vi "Read for Get Command.vi"(8 "error in (no error)":errorcluster, 10 "Control Name":string, 11 "TCP Network Connection in":refnum<k5>) -> (0 "error out":errorcluster)   [LabVIEW 2019]
doc: "Author: Scott Hannahs <sth@magnet.fsu.edu>\nCopyright 2018 Florida State University, All rights reserved."
uses:
  SCH Data Controls/FPGA Magnet Config.ctl
  SCH Data Controls/SCH Data 2 RT.ctl
  <vilib>/Utility/error.llb/Error Cluster From Error Code.vi
  TCP Functions/TCP Read Length and Value (I16).vi
  TCP Functions/TCP Read Length and Value (U16).vi
  TCP Functions/TCP Read Length and Value (I32).vi
  TCP Functions/TCP Read Length and Value (U32).vi
  TCP Functions/TCP Read Length and Value (Double).vi
  TCP Functions/TCP Read Length and Value (STR).vi
  TCP Functions/TCP Read Length and Value (Bool).vi
  TCP Functions/TCP Read Length and Value (DateStamp).vi
  TCP Functions/TCP Read Length and Value (Variant).vi
  TCP Functions/TCP Read Length and Value (Array I16).vi
  TCP Functions/TCP Read Length and Value (Array Dbl).vi
  TCP Functions/TCP Read Length and Value (2D Array Dbl).vi
  <vilib>/ErrorRing/Error Ring.xnode
  <vilib>/Utility/Data Type/NI_Data Type.lvlib
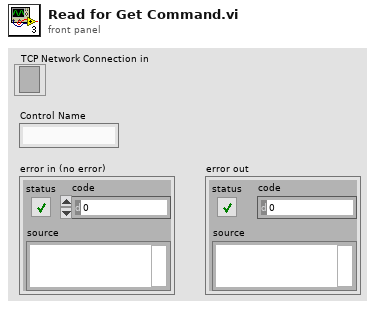
[diagram p1: front panel]
types:
  T1 = typedef "NI_Data Type.lvlib/Data Type.ctl" = enum8{"Invalid Type", "Void", "I8", "I16", "I32", "I64", "U8", "U16", "U32", "U64", "Single Float", "Double Float", "Extended Float", "Single Complex", "Double Complex", "Extended Complex", "Enum U8", "Enum U16", "Enum U32", "Enum U64", "Single Float With Unit", "Double Float With Unit", "Extended Float With Unit", "Single Complex with Unit", "Double Complex with Unit", "Extended Complex with Unit", "Boolean", "String", "Path", "Picture", "Tag", "Array", "Cluster", "Variant", "LV Variant", "Waveform", "Timestamp", "Digital Waveform", "Digital Data", "ExpressData", "Refnum", "External Data", "VI", "Poly VI", "LabVIEW Class Instance", "Fixed Point", "Set Collection", "Map Collection"}
  T2 = typedef "FPGA Magnet Config.ctl" = cluster{"#Coils":u32, "Coil Inductances":T3[], "Max Coil Currents":T3[], "Max Coil Volt Dev":T3[], "Coil A Coefficients":T3[], "Coil B Coefficients":T3[], "Coil C Coefficients":T3[], "Coil D Coefficients":T3[], "Max Coil Temp":T3[], " Pressure Range":T3[], "Temp Coef":T3[], "Offsets":T3[], "Scale Factors":T3[]}
  T3 = typedef "SCH Data 2 RT.ctl" = fxp<+/-,38,12>
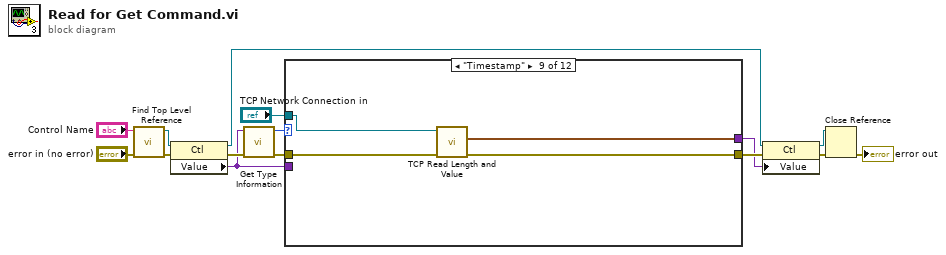
[diagram p0: block diagram]
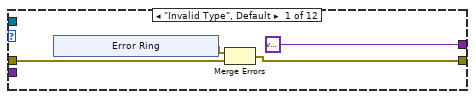
[diagram p2: hidden frame]
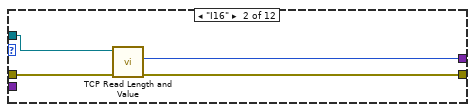
[diagram p3: hidden frame]
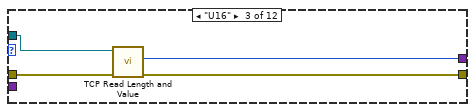
[diagram p4: hidden frame]
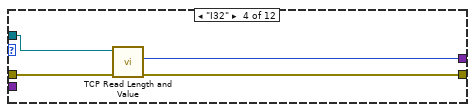
[diagram p5: hidden frame]
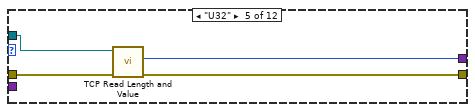
[diagram p6: hidden frame]
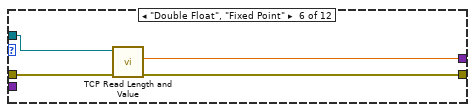
[diagram p7: hidden frame]
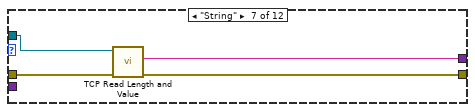
[diagram p8: hidden frame]
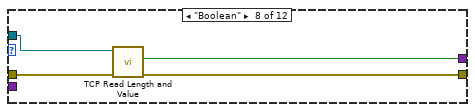
[diagram p9: hidden frame]
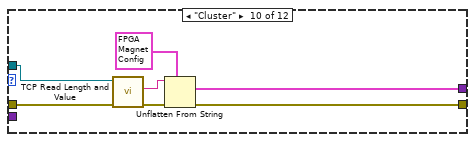
[diagram p10: hidden frame]
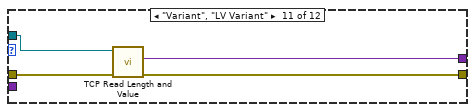
[diagram p11: hidden frame]
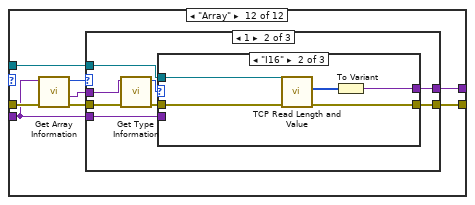
[diagram p12: hidden frame]
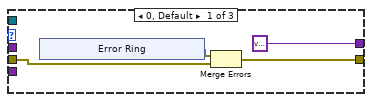
[diagram p13: hidden frame]
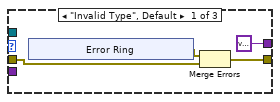
[diagram p14: hidden frame]
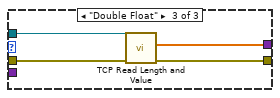
[diagram p15: hidden frame]
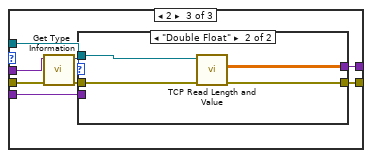
[diagram p16: hidden frame]
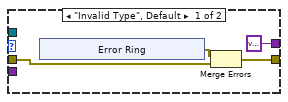
[diagram p17: hidden frame]
diagram:
  n1 = call "Find Top Level Reference.vi"("error in (no error)"="error in (no error)", "String"="Control Name") -> ("error out"=w11:errorcluster, "Ctl Refnum"=w10:refnum<vi>)  [unwired: 8 in]
  n2 = property class="Ctl"(reference=w10, error in=w11) -> (reference out=w1:refnum<vi>, error out=w12:errorcluster, "Value"=w5:variant)
  n3 = call <vilib>:"Get Type Information.vi"("error in (no error)"=w12, "variant"=w5) -> ("error out"=w6:errorcluster, "type"=w7:T1)  [unwired: 5 in, 3 out]
  n4 = case shown="\"Timestamp\"" w7 {
    tunnel: w5 -> [_ _ _ _ _ _ _ _ _ _ _ w69]
    tunnel: "TCP Network Connection in" -> [_ w26 w29 w36 w38 w43 w45 w50 w54 w63 w65 w75]
    tunnel: w6 -> [w19 w25 w32 w33 w37 w41 w46 w49 w53 w59 w64 w71]
    tunnel: [w18 w28 w31 w34 w40 w44 w47 w52 w56 w57 w67 w74] -> w3
    tunnel: [variant ("Variant") w27 w30 w35 w39 w42 w48 w51 w55 w60 w66 w68] -> w2
    frame "Invalid Type", Default {
      n5 = xnode "Error Ring"() -> ("error out"=w17:errorcluster)
      n6 = Merge Errors(w17, w19) -> (w18:errorcluster)
    }
    frame "I16" {
      n7 = call-poly "TCP Read Length and Value.vi"("error in (no error)"=w25, "TCP Network Connection in"=w26) -> ("error out"=w28:errorcluster, "Output"=w27:i16)  [unwired: 7 in, 1 out]
    }
    frame "U16" {
      n8 = call-poly "TCP Read Length and Value.vi"("error in (no error)"=w32, "TCP Network Connection in"=w29) -> ("error out"=w31:errorcluster, "Output"=w30:u16)  [unwired: 7 in, 1 out]
    }
    frame "I32" {
      n9 = call-poly "TCP Read Length and Value.vi"("error in (no error)"=w33, "TCP Network Connection in"=w36) -> ("error out"=w34:errorcluster, "Output"=w35:i32)  [unwired: 7 in, 1 out]
    }
    frame "U32" {
      n10 = call-poly "TCP Read Length and Value.vi"("error in (no error)"=w37, "TCP Network Connection in"=w38) -> ("error out"=w40:errorcluster, "Output"=w39:u32)  [unwired: 7 in, 1 out]
    }
    frame "Double Float", "Fixed Point" {
      n11 = call-poly "TCP Read Length and Value.vi"("error in (no error)"=w41, "TCP Network Connection in"=w43) -> ("error out"=w44:errorcluster, "Output"=w42:dbl)  [unwired: 7 in, 1 out]
    }
    frame "String" {
      n12 = call-poly "TCP Read Length and Value.vi"("error in (no error)"=w46, "TCP Network Connection in"=w45) -> ("error out"=w47:errorcluster, "Output"=w48:string)  [unwired: 7 in, 1 out]
    }
    frame "Boolean" {
      n13 = call-poly "TCP Read Length and Value.vi"("error in (no error)"=w49, "TCP Network Connection in"=w50) -> ("error out"=w52:errorcluster, "Output"=w51:bool)  [unwired: 7 in, 1 out]
    }
    frame "Timestamp" {
      n14 = call-poly "TCP Read Length and Value.vi"("error in (no error)"=w53, "TCP Network Connection in"=w54) -> ("error out"=w56:errorcluster, "Output"=w55:timestamp)  [unwired: 7 in, 1 out]
    }
    frame "Cluster" {
      n15 = call-poly "TCP Read Length and Value.vi"("error in (no error)"=w59, "TCP Network Connection in"=w63) -> ("error out"=w58:errorcluster, "Output"=w62:string)  [unwired: 7 in, 1 out]
      n16 = Unflatten From String(type=T2 {"#Coils"=4, "Coil Inductances"=[0.10000002384185791, 0.3999999761581421, 0.6000000238418579, 1.199999988079071], "Max Coil Currents"=[19.899999976158142, 19.899999976158142, 19.899999976158142, 19.899999976158142], "Max Coil Volt Dev"=[1.800000011920929, 2.100000023841858, 3.100000023841858, 2.600000023841858], "Coil A Coefficients"=[0.8209999799728394, 0.00010001659393310547, 5.960464477539063e-08], "Coil B Coefficients"=[0.8999999761581421, 0.00019997358322143555, 2.9802322387695312e-06], "Coil C Coefficients"=[1.100000023841858, 0.0, 0.0], "Coil D Coefficients"=[1.0, 0.0009999871253967285, 0.0], "Max Coil Temp"=[100.0, 80.0, 80.0, 60.0], " Pressure Range"=[29.30000001192093, 32.30000001192093], "Temp Coef"=[0.0031999945640563965, 0.0031999945640563965, 0.0029000043869018555, 0.004100024700164795], "Offsets"=[0.0, 0.0, -5.0, -5.0, 0.0, 0.0, 0.0, 0.0, 0.0, 0.0, 0.0, 0.0, 0.0, 0.0, 0.0], "Scale Factors"=[20.0, 20.0, 4.2670000195503235, 4.269999980926514, 4.0, 1.0, 1.0, 1.0, 1.0, 1.0, -2.0, 30.08600002527237, 29.861999988555908, 35.50199997425079, 35.56999999284744]} ("Magnet Configuration Data"), binary string=w62, error in (no error)=w58) -> (value=w60:T2, error out=w57:errorcluster)  [unwired: 2 in, 1 out]
    }
    frame "Variant", "LV Variant" {
      n17 = call-poly "TCP Read Length and Value.vi"("error in (no error)"=w64, "TCP Network Connection in"=w65) -> ("error out"=w67:errorcluster, "Output"=w66:variant)  [unwired: 7 in, 1 out]
    }
    frame "Array" {
      n18 = call <vilib>:"Get Array Information.vi"("error in (no error)"=w71, "variant"=w69) -> ("error out"=w70:errorcluster, "array element data type"=w72:variant, "number of dimensions"=w73:i32)  [unwired: 6 in, 1 out]
      n19 = case shown="1" w73 {
        tunnel: w69 -> [_ w92 w118]
        tunnel: w75 -> [_ w91 w117]
        tunnel: w70 -> [w78 w87 w113]
        tunnel: [w77 w90 w116] -> w74
        tunnel: w72 -> [_ w89 w115]
        tunnel: [variant ("Variant") w85 w111] -> w68
        frame 0, Default {
          n20 = xnode "Error Ring"() -> ("error out"=w79:errorcluster)
          n21 = Merge Errors(w79, w78) -> (w77:errorcluster)
        }
        frame 1 {
          n22 = call <vilib>:"Get Type Information.vi"("error in (no error)"=w87, "variant"=w89) -> ("error out"=w86:errorcluster, "type"=w88:T1)  [unwired: 5 in, 3 out]
          n23 = case shown="\"I16\"" w88 {
            tunnel: w92 -> [_ _ _]
            tunnel: w91 -> [_ w106 w108]
            tunnel: w86 -> [w95 w105 w107]
            tunnel: [w94 w104 w110] -> w90
            tunnel: [variant ("Variant") w102 w109] -> w85
            frame "Invalid Type", Default {
              n24 = xnode "Error Ring"() -> ("error out"=w96:errorcluster)
              n25 = Merge Errors(w96, w95) -> (w94:errorcluster)
            }
            frame "I16" {
              n26 = call-poly "TCP Read Length and Value.vi"("error in (no error)"=w105, "TCP Network Connection in"=w106) -> ("error out"=w104:errorcluster, "Output"=w103:i16[])  [unwired: 7 in, 1 out]
              n27 = To Variant(anything=w103) -> (Variant=w102:variant)
            }
            frame "Double Float" {
              n28 = call-poly "TCP Read Length and Value.vi"("error in (no error)"=w107, "TCP Network Connection in"=w108) -> ("error out"=w110:errorcluster, "Output"=w109:dbl[])  [unwired: 7 in, 1 out]
            }
          }
        }
        frame 2 {
          n29 = call <vilib>:"Get Type Information.vi"("error in (no error)"=w113, "variant"=w115) -> ("error out"=w112:errorcluster, "type"=w114:T1)  [unwired: 5 in, 3 out]
          n30 = case shown="\"Double Float\"" w114 {
            tunnel: w118 -> [_ _]
            tunnel: w117 -> [_ w130]
            tunnel: w112 -> [w121 w128]
            tunnel: [w120 w129] -> w116
            tunnel: [variant ("Variant") w131] -> w111
            frame "Invalid Type", Default {
              n31 = xnode "Error Ring"() -> ("error out"=w122:errorcluster)
              n32 = Merge Errors(w122, w121) -> (w120:errorcluster)
            }
            frame "Double Float" {
              n33 = call-poly "TCP Read Length and Value.vi"("error in (no error)"=w128, "TCP Network Connection in"=w130) -> ("error out"=w129:errorcluster, "Array"=w131:dbl[][])  [unwired: 7 in, 1 out]
            }
          }
        }
      }
    }
  }
  n34 = property class="Ctl"(reference=w1, error in=w3, "Value"=w2) -> (reference out=w14:refnum<vi>, error out=w15:errorcluster)
  n35 = Close Reference(reference=w14, error in (no error)=w15) -> (error out=→"error out":errorcluster)
